vi "subGetItemInfosFromProjectRef.vi"(8 "error in (no error)":errorcluster, 11 "SolutionBuilder in":refnum<class "SolutionBuilder.lvclass">) -> (0 "error out":errorcluster, 3 "SolutionBuilder out":refnum<class "SolutionBuilder.lvclass">)   [LabVIEW 2020, in "SolutionBuilder.lvlib" / "SolutionBuilder.lvclass"]
uses:
  SolutionBuilder.lvclass
  SolutionBuilder.lvclass/SolutionBuilder.ctl
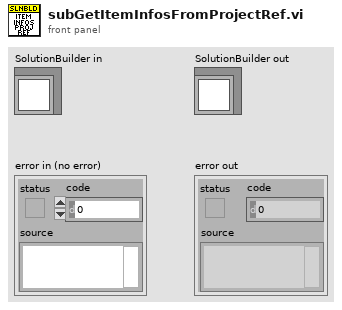
[diagram p1: front panel]
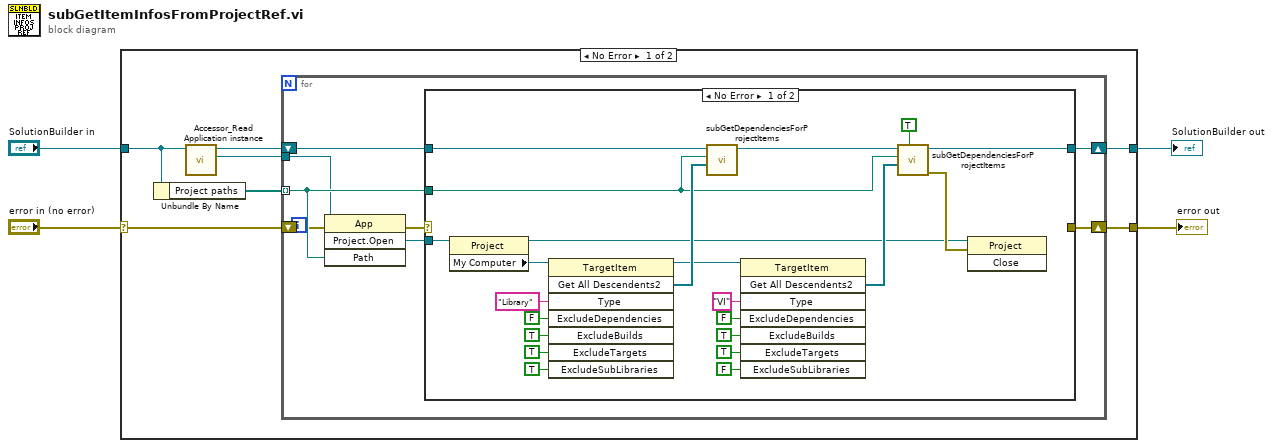
[diagram p0: block diagram]
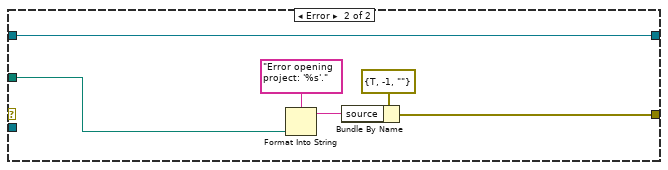
[diagram p2: hidden frame]
diagram:
  n1 = case shown="No Error" "error in (no error)" {
    selector: "error in (no error)" -> [w5 w48]
    tunnel: [w10 w49] -> w4
    tunnel: "SolutionBuilder in" -> [w9 w49]
    tunnel: [w6 w48] -> w1
    frame No Error {
      n2 = Unbundle By Name(w9) -> ("Project paths"=w11:path[])
      n3 = call "Accessor_Read Application instance.vi"("SolutionBuilder in"=w9) -> ("App instance"=w7:refnum<vi>, "SolutionBuilder out"=w8:refnum<class "SolutionBuilder.lvclass">)  [unwired: 8 in, 1 out]
      n4 = for {
        tunnel: w11 -> [w18] mode=indexing
        shift-right: [w17] -> w10
        shift-left: w8 -> [w19]
        tunnel: w7 -> [w14]
        shift-right: [w13] -> w6
        shift-left: w5 -> [w12]
        n5 = invoke class="App" method="Project.Open"(reference=w14, error in=w12, "Path"=w18) -> (error out=w15:errorcluster, "Project:Open"=w16:refnum<vi>)  [unwired: 1 in, 2 out]
        n6 = case shown="No Error" w15 {
          tunnel: w19 -> [w30 w47]
          tunnel: w18 -> [w26 w46]
          tunnel: [w24 w47] -> w17
          tunnel: w16 -> [w21 _]
          tunnel: [_ w42] -> w13
          frame No Error {
            n7 = property class="Project"(reference=w21) -> (reference out=w20:refnum<vi>, "My Computer"=w31:refnum<vi>)  [unwired: 1 in, 1 out]
            n8 = invoke class="TargetItem" method="Get All Descendents2"(reference=w31, "Type"="Library", "ExcludeDependencies"=FALSE, "ExcludeBuilds"=TRUE, "ExcludeTargets"=TRUE, "ExcludeSubLibraries"=TRUE) -> (reference out=w23:refnum<vi>, "Get All Descendents2"=w29:refnum<vi>[])  [unwired: 2 in, 6 out]
            n9 = call "subGetDependenciesForProjectItems.vi"("Dependents"=w29, "Owning project"=w26, "SolutionBuilder in"=w30) -> ("SolutionBuilder out"=w28:refnum<class "SolutionBuilder.lvclass">)  [unwired: 7 in, 1 out]
            n10 = invoke class="TargetItem" method="Get All Descendents2"(reference=w23, "Type"="VI", "ExcludeDependencies"=FALSE, "ExcludeBuilds"=TRUE, "ExcludeTargets"=TRUE, "ExcludeSubLibraries"=FALSE) -> ("Get All Descendents2"=w25:refnum<vi>[])  [unwired: 2 in, 7 out]
            n11 = call "subGetDependenciesForProjectItems.vi"("Shallow check"=TRUE, "Dependents"=w25, "Owning project"=w26, "SolutionBuilder in"=w28) -> ("error out"=w22:errorcluster, "SolutionBuilder out"=w24:refnum<class "SolutionBuilder.lvclass">)  [unwired: 6 in]
            n12 = invoke class="Project" method="Close"(reference=w20, error in=w22) -> ()  [unwired: 1 in, 3 out]
          }
          frame Error {
            n13 = Format Into String(format string="Error opening project: '%s'.", w46) -> (resulting string=w44:string)  [unwired: 2 in, 1 out]
            n14 = Bundle By Name(cluster=errorcluster {"status"=TRUE, "code"=-1, "source"=""} ("t"), "source"=w44) -> (w42:errorcluster)
          }
        }
      }
    }
    frame Error {
    }
  }
  "SolutionBuilder out" <- w4
  "error out" <- w1
